vi "Examine cluster elements.vi"() -> ()   [LabVIEW 2013]
panel:
  out "Array 2":cluster{string[]}[](array[cluster])
  out "Array":string[](array[string])
  in  "Best Pattern (0) Distance data (1 to X) cluster (X+1) output":string[][](array[string])
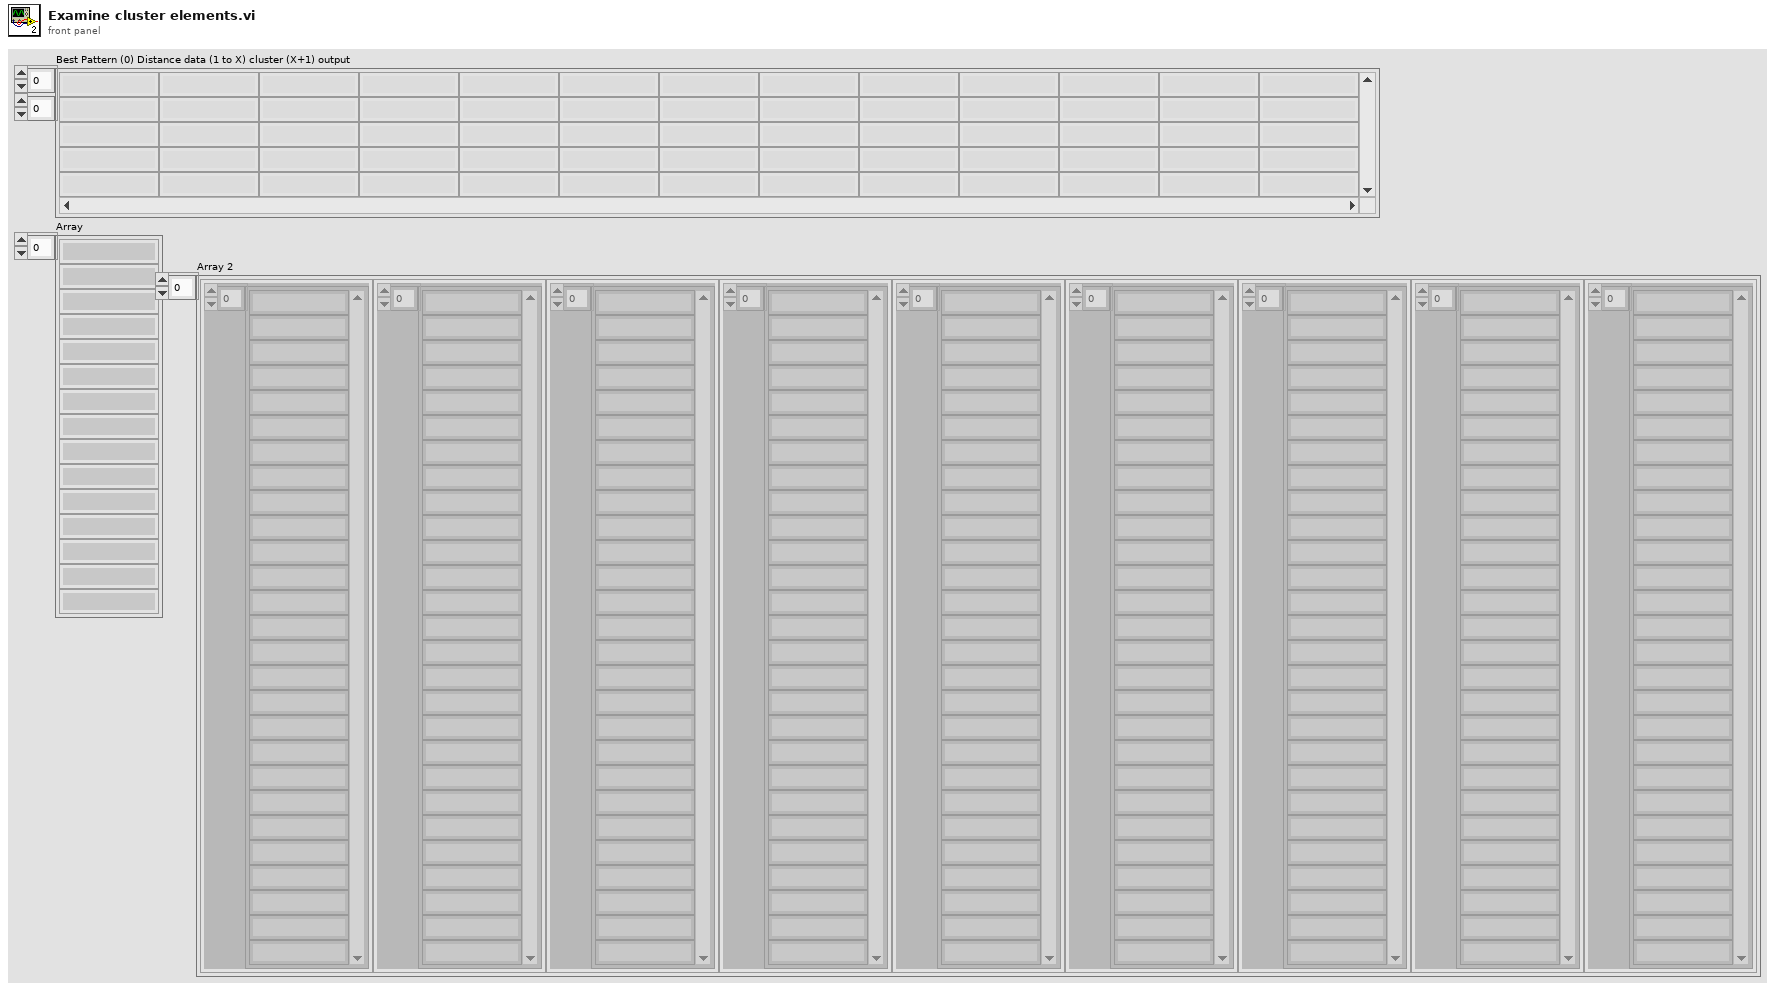
[diagram p1: front panel]
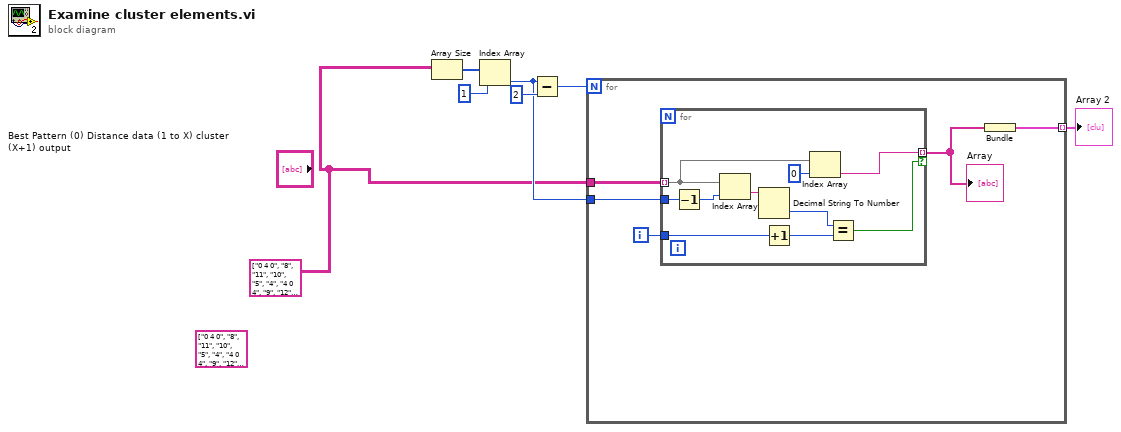
[diagram p0: block diagram]
diagram:
  w1 = string[][] [["0 4 0", "8", "11", "10", "5", "4"], ["4 0 4", "9", "12", "8", "6", "4"], ["0 4 0", "8", "11", "10", "5", "4"], ["4 0 4", "9", "12", "8", "6", "4"], ["0 4 0", "8", "11", "10", "5", "4"], ["4 0 4", "9", "12", "8", "6", "4"], ["0 4 0", "8", "11", "10", "5", "4"], ["4 0 -2", "10", "8", "7", "10", "3"], ["0 -2 3", "13", "3", "8", "12", "2"], ["-2 3 0", "16", "8", "8", "14", "0"], ["3 0 3", "13", "9", "6", "10", "3"], ["0 3 0", "12", "7", "9", "9", "2"], ["3 0 4", "11", "11", "6", "7", "3"], ["0 4 0", "8", "11", "10", "5", "4"], ["-2 0 1", "8", "7", "2", "11", "3"], ["0 1 0", "2", "9", "9", "7", "1"], ["1 0 -4", "4", "11", "7", "7", "1"], ["0 -4 4", "6", "14", "12", "0", "4"], ["-2 2 0", "12", "6", "7", "16", "2"], ["2 0 -1", "8", "8", "2", "11", "3"], ["0 -1 -4", "4", "9", "7", "8", "1"], ["-1 -4 1", "6", "14", "12", "5", "4"], ["-4 1 0", "4", "14", "13", "8", "1"], ["1 0 3", "9", "10", "8", "9", "3"], ["0 3 0", "12", "7", "9", "9", "2"], ["-1 0 -1", "7", "7", "3", "9", "3"], ["0 -1 2", "7", "5", "6", "12", "2"], ["0 -1 1", "5", "8", "6", "10", "1"], ["-1 1 0", "4", "11", "11", "9", "1"], ["1 0 4", "7", "12", "8", "6", "4"], ["0 4 0", "8", "11", "10", "5", "4"], ["4 0 3", "11", "10", "8", "9", "3"], ["0 3 -2", "14", "6", "11", "11", "2"], ["3 -2 0", "15", "5", "6", "15", "2"], ["-2 0 -2", "11", "5", "3", "12", "3"], ["0 -2 3", "13", "3", "8", "12", "2"], ["-2 3 -2", "18", "7", "10", "16", "2"], ["3 -2 0", "15", "5", "6", "15", "2"], ["-2 0 4", "10", "9", "4", "8", "3"], ["0 4 0", "8", "11", "10", "5", "4"], ["4 0 -2", "10", "8", "7", "10", "3"], ["0 -2 2", "11", "0", "6", "14", "2"], ["2 -1 0", "9", "10", "6", "13", "3"], ["-1 0 4", "8", "10", "7", "5", "4"], ["0 4 0", "8", "11", "10", "5", "4"], ["4 0 2", "9", "7", "6", "11", "3"], ["0 2 0", "8", "5", "8", "11", "2"], ["2 0 -2", "10", "7", "5", "11", "3"], ["0 -2 0", "10", "2", "5", "11", "2"], ["1 -1 0", "7", "11", "8", "12", "1"], ["-1 0 3", "10", "8", "7", "8", "3"], ["0 3 0", "12", "7", "9", "9", "2"], ["3 0 -4", "8", "10", "5", "8", "3"], ["0 -4 4", "6", "14", "12", "0", "4"], ["-4 4 -4", "8", "18", "16", "5", "4"], ["4 -4 0", "8", "15", "12", "5", "4"], ["2 -1 0", "9", "10", "6", "13", "3"], ["-1 0 3", "10", "8", "7", "8", "3"], ["0 3 -2", "14", "6", "11", "11", "2"], ["3 -2 0", "15", "5", "6", "15", "2"], ["-2 0 -3", "11", "8", "5", "10", "3"], ["0 -3 0", "10", "9", "9", "7", "4"], ["-3 0 3", "12", "8", "7", "8", "3"], ["0 3 0", "12", "7", "9", "9", "2"], ["3 0 -3", "12", "10", "7", "9", "3"], ["0 -3 0", "10", "9", "9", "7", "4"], ["0 4 0", "8", "11", "10", "5", "4"], ["4 0 4", "9", "12", "8", "6", "4"], ["0 4 -4", "6", "13", "12", "4", "4"], ["4 -4 1", "7", "16", "13", "6", "4"], ["-4 1 -1", "4", "14", "12", "10", "1"], ["1 -1 0", "7", "11", "8", "12", "1"], ["-1 0 -3", "9", "9", "8", "7", "4"], ["0 -3 0", "10", "9", "9", "7", "4"], ["-3 0 1", "8", "8", "5", "8", "3"], ["0 1 -4", "0", "11", "11", "6", "1"], ["1 -4 1", "5", "16", "13", "6", "1"], ["-4 1 0", "4", "14", "13", "8", "1"], ["1 0 4", "7", "12", "8", "6", "4"], ["0 4 0", "8", "11", "10", "5", "4"], ["4 0 -4", "6", "11", "7", "7", "1"], ["0 -4 0", "5", "11", "9", "2", "4"], ["-4 0 -4", "5", "12", "8", "5", "0"], ["0 -4 4", "6", "14", "12", "0", "4"], ["-4 4 -4", "8", "18", "16", "5", "4"], ["4 -4 1", "7", "16", "13", "6", "4"], ["0 -4 1", "4", "12", "10", "3", "4"], ["-4 1 0", "4", "14", "13", "8", "1"], ["1 0 -4", "4", "11", "7", "7", "1"], ["0 -4 4", "6", "14", "12", "0", "4"], ["0 4 0", "8", "11", "10", "5", "4"], ["4 0 -2", "10", "8", "7", "10", "3"], ["0 -2 2", "11", "0", "6", "14", "2"], ["-2 2 -2", "14", "5", "9", "18", "2"], ["2 -2 2", "14", "3", "7", "18", "2"], ["-2 2 -2", "14", "5", "9", "18", "2"], ["2 -2 2", "14", "3", "7", "18", "2"], ["-2 2 -1", "12", "6", "6", "18", "0"], ["2 -1 0", "9", "10", "6", "13", "3"], ["-1 0 4", "8", "10", "7", "5", "4"], ["0 4 0", "8", "11", "10", "5", "4"], ["4 0 2", "9", "7", "6", "11", "3"], ["0 2 0", "8", "5", "8", "11", "2"], ["2 0 4", "9", "11", "6", "7", "3"], ["0 4 0", "8", "11", "10", "5", "4"], ["4 0 2", "9", "7", "6", "11", "3"], ["0 2 -2", "10", "4", "10", "13", "2"], ["2 -2 0", "13", "5", "6", "15", "2"], ["-2 0 4", "10", "9", "4", "8", "3"], ["1 0 -1", "6", "9", "4", "10", "3"], ["0 -1 0", "6", "7", "5", "9", "3"], ["-1 0 -1", "7", "7", "3", "9", "3"], ["0 -1 0", "6", "7", "5", "9", "3"], ["-1 0 1", "6", "8", "5", "8", "3"], ["0 1 -1", "2", "9", "8", "9", "1"], ["-2 2 -2", "14", "5", "9", "18", "2"], ["2 -2 3", "16", "6", "9", "16", "2"], ["1 0 -1", "6", "9", "4", "10", "3"], ["0 -1 0", "6", "7", "5", "9", "3"], ["-1 0 -1", "7", "7", "3", "9", "3"], ["0 -1 2", "7", "5", "6", "12", "2"], ["-1 2 0", "10", "7", "10", "13", "2"], ["2 0 2", "9", "6", "4", "12", "3"], ["0 2 -2", "10", "4", "10", "13", "2"], ["2 -2 0", "13", "5", "6", "15", "2"], ["-2 0 -4", "7", "8", "3", "9", "3"], ["0 -4 0", "5", "11", "9", "2", "4"], ["-2 2 0", "12", "6", "7", "16", "2"], ["2 0 3", "11", "9", "6", "10", "3"], ["0 3 -2", "14", "6", "11", "11", "2"], ["3 -2 2", "16", "3", "7", "18", "2"], ["1 -1 0", "7", "11", "8", "12", "1"], ["-1 0 3", "10", "8", "7", "8", "3"], ["0 4 0", "8", "11", "10", "5", "4"], ["-2 0 1", "8", "7", "2", "11", "3"], ["0 1 -4", "0", "11", "11", "6", "1"], ["1 -4 0", "6", "15", "12", "5", "4"], ["-4 0 -3", "9", "12", "10", "6", "4"], ["0 -3 0", "10", "9", "9", "7", "4"], ["1 0 -1", "6", "9", "4", "10", "3"], ["0 -1 2", "7", "5", "6", "12", "2"], ["-1 2 -1", "10", "7", "9", "15", "2"], ["2 -1 1", "8", "11", "7", "14", "3"], ["-1 1 -4", "2", "13", "13", "8", "1"], ["-2 0 -1", "9", "6", "0", "12", "3"], ["0 -1 1", "5", "8", "6", "10", "1"], ["0 3 0", "12", "7", "9", "9", "2"], ["3 0 3", "13", "9", "6", "10", "3"], ["0 3 0", "12", "7", "9", "9", "2"], ["3 0 3", "13", "9", "6", "10", "3"], ["0 3 -2", "14", "6", "11", "11", "2"], ["-4 0 -4", "5", "12", "8", "5", "0"], ["0 -4 4", "6", "14", "12", "0", "4"], ["0 4 0", "8", "11", "10", "5", "4"], ["4 0 -4", "6", "11", "7", "7", "1"], ["0 -4 0", "5", "11", "9", "2", "4"], ["-4 0 -4", "5", "12", "8", "5", "0"], ["-2 2 0", "12", "6", "7", "16", "2"], ["2 0 4", "9", "11", "6", "7", "3"], ["0 4 -4", "6", "13", "12", "4", "4"], ["4 -4 0", "8", "15", "12", "5", "4"], ["-4 0 2", "8", "8", "7", "9", "3"], ["0 2 -2", "10", "4", "10", "13", "2"]] ("Best Pattern (0) Distance data (1 to X) cluster (X+1) output")
  (unwired) string[][] [["0 4 0", "8", "11", "10", "5", "4"], ["4 0 4", "9", "12", "8", "6", "4"], ["0 4 0", "8", "11", "10", "5", "4"], ["4 0 4", "9", "12", "8", "6", "4"], ["0 4 0", "8", "11", "10", "5", "4"], ["4 0 4", "9", "12", "8", "6", "4"], ["0 4 0", "8", "11", "10", "5", "4"], ["4 0 -2", "10", "8", "7", "10", "3"], ["0 -2 3", "13", "3", "8", "12", "2"], ["-2 3 0", "16", "8", "8", "14", "0"], ["3 0 3", "13", "9", "6", "10", "3"], ["0 3 0", "12", "7", "9", "9", "2"], ["3 0 4", "11", "11", "6", "7", "3"], ["0 4 0", "8", "11", "10", "5", "4"], ["-2 0 1", "8", "7", "2", "11", "3"], ["0 1 0", "2", "9", "9", "7", "1"], ["1 0 -4", "4", "11", "7", "7", "1"], ["0 -4 4", "6", "14", "12", "0", "4"], ["-2 2 0", "12", "6", "7", "16", "2"], ["2 0 -1", "8", "8", "2", "11", "3"], ["0 -1 -4", "4", "9", "7", "8", "1"], ["-1 -4 1", "6", "14", "12", "5", "4"], ["-4 1 0", "4", "14", "13", "8", "1"], ["1 0 3", "9", "10", "8", "9", "3"], ["0 3 0", "12", "7", "9", "9", "2"], ["-1 0 -1", "7", "7", "3", "9", "3"], ["0 -1 2", "7", "5", "6", "12", "2"], ["0 -1 1", "5", "8", "6", "10", "1"], ["-1 1 0", "4", "11", "11", "9", "1"], ["1 0 4", "7", "12", "8", "6", "4"], ["0 4 0", "8", "11", "10", "5", "4"], ["4 0 3", "11", "10", "8", "9", "3"], ["0 3 -2", "14", "6", "11", "11", "2"], ["3 -2 0", "15", "5", "6", "15", "2"], ["-2 0 -2", "11", "5", "3", "12", "3"], ["0 -2 3", "13", "3", "8", "12", "2"], ["-2 3 -2", "18", "7", "10", "16", "2"], ["3 -2 0", "15", "5", "6", "15", "2"], ["-2 0 4", "10", "9", "4", "8", "3"], ["0 4 0", "8", "11", "10", "5", "4"], ["4 0 -2", "10", "8", "7", "10", "3"], ["0 -2 2", "11", "0", "6", "14", "2"], ["2 -1 0", "9", "10", "6", "13", "3"], ["-1 0 4", "8", "10", "7", "5", "4"], ["0 4 0", "8", "11", "10", "5", "4"], ["4 0 2", "9", "7", "6", "11", "3"], ["0 2 0", "8", "5", "8", "11", "2"], ["2 0 -2", "10", "7", "5", "11", "3"], ["0 -2 0", "10", "2", "5", "11", "2"], ["1 -1 0", "7", "11", "8", "12", "1"], ["-1 0 3", "10", "8", "7", "8", "3"], ["0 3 0", "12", "7", "9", "9", "2"], ["3 0 -4", "8", "10", "5", "8", "3"], ["0 -4 4", "6", "14", "12", "0", "4"], ["-4 4 -4", "8", "18", "16", "5", "4"], ["4 -4 0", "8", "15", "12", "5", "4"], ["2 -1 0", "9", "10", "6", "13", "3"], ["-1 0 3", "10", "8", "7", "8", "3"], ["0 3 -2", "14", "6", "11", "11", "2"], ["3 -2 0", "15", "5", "6", "15", "2"], ["-2 0 -3", "11", "8", "5", "10", "3"], ["0 -3 0", "10", "9", "9", "7", "4"], ["-3 0 3", "12", "8", "7", "8", "3"], ["0 3 0", "12", "7", "9", "9", "2"], ["3 0 -3", "12", "10", "7", "9", "3"], ["0 -3 0", "10", "9", "9", "7", "4"], ["0 4 0", "8", "11", "10", "5", "4"], ["4 0 4", "9", "12", "8", "6", "4"], ["0 4 -4", "6", "13", "12", "4", "4"], ["4 -4 1", "7", "16", "13", "6", "4"], ["-4 1 -1", "4", "14", "12", "10", "1"], ["1 -1 0", "7", "11", "8", "12", "1"], ["-1 0 -3", "9", "9", "8", "7", "4"], ["0 -3 0", "10", "9", "9", "7", "4"], ["-3 0 1", "8", "8", "5", "8", "3"], ["0 1 -4", "0", "11", "11", "6", "1"], ["1 -4 1", "5", "16", "13", "6", "1"], ["-4 1 0", "4", "14", "13", "8", "1"], ["1 0 4", "7", "12", "8", "6", "4"], ["0 4 0", "8", "11", "10", "5", "4"], ["4 0 -4", "6", "11", "7", "7", "1"], ["0 -4 0", "5", "11", "9", "2", "4"], ["-4 0 -4", "5", "12", "8", "5", "0"], ["0 -4 4", "6", "14", "12", "0", "4"], ["-4 4 -4", "8", "18", "16", "5", "4"], ["4 -4 1", "7", "16", "13", "6", "4"], ["0 -4 1", "4", "12", "10", "3", "4"], ["-4 1 0", "4", "14", "13", "8", "1"], ["1 0 -4", "4", "11", "7", "7", "1"], ["0 -4 4", "6", "14", "12", "0", "4"], ["0 4 0", "8", "11", "10", "5", "4"], ["4 0 -2", "10", "8", "7", "10", "3"], ["0 -2 2", "11", "0", "6", "14", "2"], ["-2 2 -2", "14", "5", "9", "18", "2"], ["2 -2 2", "14", "3", "7", "18", "2"], ["-2 2 -2", "14", "5", "9", "18", "2"], ["2 -2 2", "14", "3", "7", "18", "2"], ["-2 2 -1", "12", "6", "6", "18", "0"], ["2 -1 0", "9", "10", "6", "13", "3"], ["-1 0 4", "8", "10", "7", "5", "4"], ["0 4 0", "8", "11", "10", "5", "4"], ["4 0 2", "9", "7", "6", "11", "3"], ["0 2 0", "8", "5", "8", "11", "2"], ["2 0 4", "9", "11", "6", "7", "3"], ["0 4 0", "8", "11", "10", "5", "4"], ["4 0 2", "9", "7", "6", "11", "3"], ["0 2 -2", "10", "4", "10", "13", "2"], ["2 -2 0", "13", "5", "6", "15", "2"], ["-2 0 4", "10", "9", "4", "8", "3"], ["1 0 -1", "6", "9", "4", "10", "3"], ["0 -1 0", "6", "7", "5", "9", "3"], ["-1 0 -1", "7", "7", "3", "9", "3"], ["0 -1 0", "6", "7", "5", "9", "3"], ["-1 0 1", "6", "8", "5", "8", "3"], ["0 1 -1", "2", "9", "8", "9", "1"], ["-2 2 -2", "14", "5", "9", "18", "2"], ["2 -2 3", "16", "6", "9", "16", "2"], ["1 0 -1", "6", "9", "4", "10", "3"], ["0 -1 0", "6", "7", "5", "9", "3"], ["-1 0 -1", "7", "7", "3", "9", "3"], ["0 -1 2", "7", "5", "6", "12", "2"], ["-1 2 0", "10", "7", "10", "13", "2"], ["2 0 2", "9", "6", "4", "12", "3"], ["0 2 -2", "10", "4", "10", "13", "2"], ["2 -2 0", "13", "5", "6", "15", "2"], ["-2 0 -4", "7", "8", "3", "9", "3"], ["0 -4 0", "5", "11", "9", "2", "4"], ["-2 2 0", "12", "6", "7", "16", "2"], ["2 0 3", "11", "9", "6", "10", "3"], ["0 3 -2", "14", "6", "11", "11", "2"], ["3 -2 2", "16", "3", "7", "18", "2"], ["1 -1 0", "7", "11", "8", "12", "1"], ["-1 0 3", "10", "8", "7", "8", "3"], ["0 4 0", "8", "11", "10", "5", "4"], ["-2 0 1", "8", "7", "2", "11", "3"], ["0 1 -4", "0", "11", "11", "6", "1"], ["1 -4 0", "6", "15", "12", "5", "4"], ["-4 0 -3", "9", "12", "10", "6", "4"], ["0 -3 0", "10", "9", "9", "7", "4"], ["1 0 -1", "6", "9", "4", "10", "3"], ["0 -1 2", "7", "5", "6", "12", "2"], ["-1 2 -1", "10", "7", "9", "15", "2"], ["2 -1 1", "8", "11", "7", "14", "3"], ["-1 1 -4", "2", "13", "13", "8", "1"], ["-2 0 -1", "9", "6", "0", "12", "3"], ["0 -1 1", "5", "8", "6", "10", "1"], ["0 3 0", "12", "7", "9", "9", "2"], ["3 0 3", "13", "9", "6", "10", "3"], ["0 3 0", "12", "7", "9", "9", "2"], ["3 0 3", "13", "9", "6", "10", "3"], ["0 3 -2", "14", "6", "11", "11", "2"], ["-4 0 -4", "5", "12", "8", "5", "0"], ["0 -4 4", "6", "14", "12", "0", "4"], ["0 4 0", "8", "11", "10", "5", "4"], ["4 0 -4", "6", "11", "7", "7", "1"], ["0 -4 0", "5", "11", "9", "2", "4"], ["-4 0 -4", "5", "12", "8", "5", "0"], ["-2 2 0", "12", "6", "7", "16", "2"], ["2 0 4", "9", "11", "6", "7", "3"], ["0 4 -4", "6", "13", "12", "4", "4"], ["4 -4 0", "8", "15", "12", "5", "4"], ["-4 0 2", "8", "8", "7", "9", "3"], ["0 2 -2", "10", "4", "10", "13", "2"]] ("Best Pattern (0) Distance data (1 to X) cluster (X+1) output")
  n1 = Array Size(array=w1) -> (size(s)=w7:i32[])
  n2 = Index Array(array=w7, index=1) -> (element=w3:i32)
  n3 = Subtract(x=w3, y=2) -> (x-y=w4:i32)
  n4 = for {
    N: w4 -> [_]
    tunnel: w1 -> [w12]
    tunnel: w3 -> [w11]
    tunnel: [w8] -> w2 mode=indexing
    i -> [w10]
    n5 = for {
      tunnel: w12 -> [w19] mode=indexing
      tunnel: w11 -> [w21]
      tunnel: w10 -> [w17]
      tunnel: [w13] -> w9 mode=indexing if=w14
      n6 = Decrement(x=w21) -> (x-1=w22:i32)
      n7 = Index Array(array=w19, index=w22) -> (element=w18:string)
      n8 = Decimal String To Number(string=w18) -> (number=w15:i32)  [unwired: 2 in, 1 out]
      n9 = Increment(x=w17) -> (x+1=w16:i32)
      n10 = Index Array(array=w19, index=0) -> (element=w13:string)
      n11 = Equal?(x=w15, y=w16) -> (x = y?=w14:bool)
    }
    "Array" <- w9
    n12 = Bundle(w9) -> (w8:cluster{string[]})  [unwired: 1 in]
  }
  "Array 2" <- w2
